vi "DB Select.vi"(6 "Select":enum16{"SelectWithQuery", "SelectWithColumn"}(ring)=enum."SelectWithColumn", 8 "error in (no error)":errorcluster, 9 "SQLTableData":T1, 10 "SQL query":string, 11 "Database in":refnum<class "SQLite Database.lvclass">) -> (0 "error out":errorcluster, 2 "data":string[][](array[string]), 3 "Database out":refnum<class "SQLite Database.lvclass">)   [LabVIEW 2023, in "HardwareAbstractionLayer_LVOOP.lvlib" / "SQLite Database.lvclass"]
uses:
  SQLite Database.lvclass
  SQLite Database.lvclass/SQLite Database.ctl
  <vilib>/addons/database/Connection.llb/Conn Execute.vi
  <vilib>/addons/database/Recordset.llb/Rec Fetch Recordset Data (R).vi
  <vilib>/addons/database/Recordset.llb/Rec Destroy - Connection.vi
  <vilib>/addons/database/NI_Database_API.lvlib
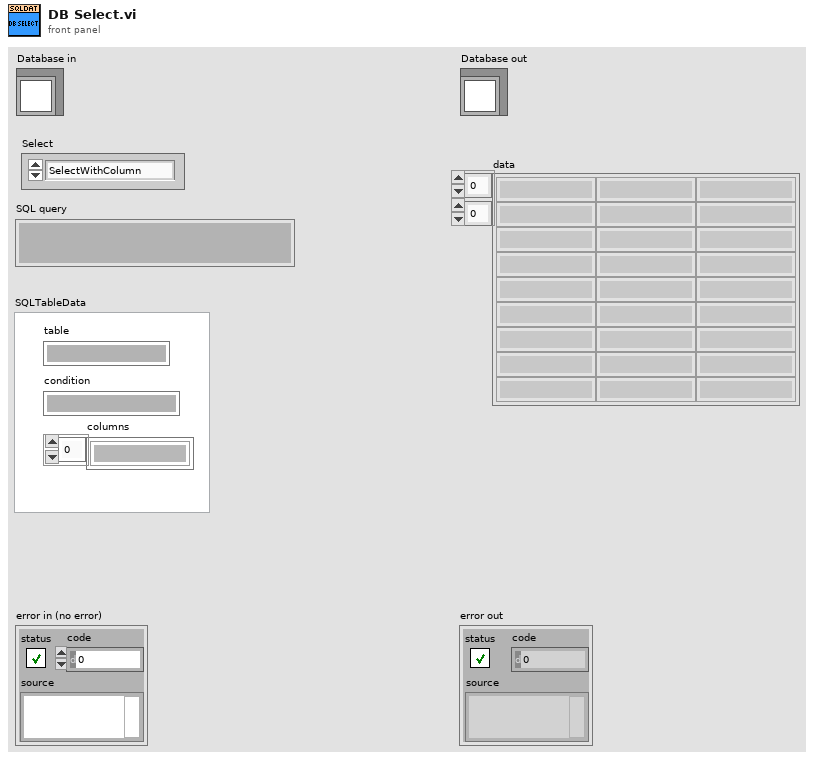
[diagram p1: front panel]
types:
  T1 = cluster{"table":string, "condition":string, "columns":string[]}
  T2 = cluster{"DataSource Name":string, "userID":string, "password":string}
  T3 = typedef "NI_Database_API.lvlib/Conn ObjectReference.ctl" = refnum<k1>
  T4 = typedef "NI_Database_API.lvlib/Rec ObjectReference.ctl" = refnum<k1>
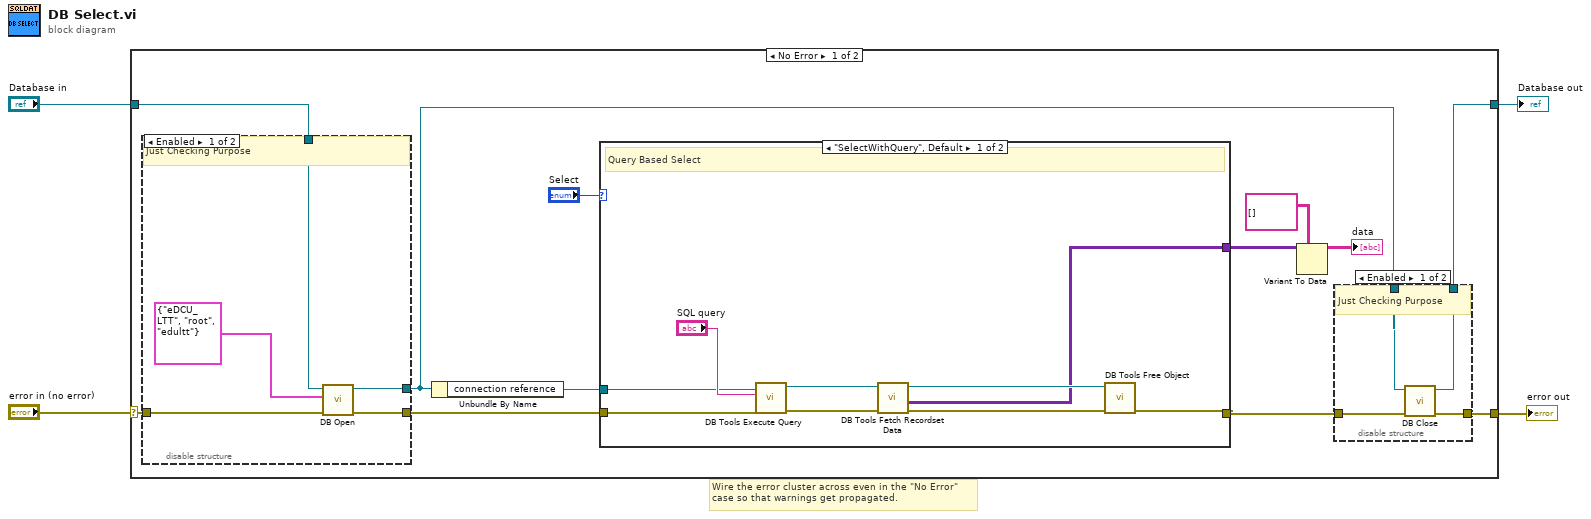
[diagram p0: block diagram]
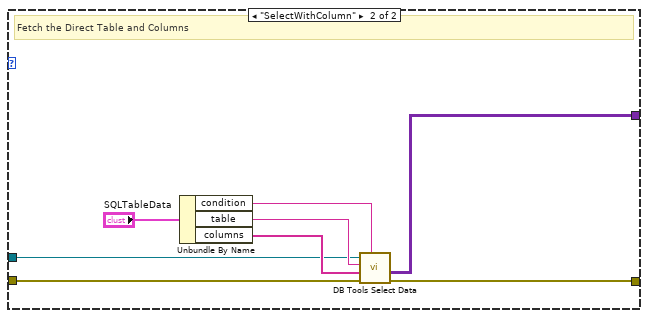
[diagram p4: hidden frame]
diagram:
  # "Wire the error cluster across even in the \"No Error\"\ncase so that warnings get propagated."
  n1 = case shown="No Error" "error in (no error)" {
    selector: "error in (no error)" -> [w11 w47]
    tunnel: [w5 w48] -> w1
    tunnel: "Database in" -> [w12 w48]
    tunnel: [w7 w47] -> w2
    frame No Error {
      n2 = disable-structure shown="Enabled" {
        disable-tunnel: w12 -> [w27 w29]
        disable-tunnel: w11 -> [w25 w28]
        disable-tunnel: [w24 w28] -> w10
        disable-tunnel: [w23 w29] -> w6
        frame Enabled {
          # "Just Checking Purpose"
          n3 = call-dynamic "DB Open.vi"("error in"=w25, "DB"=T2 {"DataSource Name"="eDCU_LTT", "userID"="root", "password"="edultt"}, "Database in"=w27) -> ("error out"=w24:errorcluster, "Database out"=w23:refnum<class "SQLite Database.lvclass">)  [unwired: 7 in]
        }
        frame Disabled {
        }
      }
      n4 = Unbundle By Name(w6) -> ("connection reference"=w9:T3)
      n5 = case shown="\"SelectWithQuery\", Default" "Select" {
        tunnel: w10 -> [w38 w46]
        tunnel: [w35 w45] -> w8
        tunnel: [w32 w44] -> w14
        tunnel: w9 -> [w30 w39]
        frame "SelectWithQuery", Default {
          # "Query Based Select"
          n6 = call-poly <vilib>:"DB Tools Execute Query.vi"("error in (no error)"=w38, "SQL query"="SQL query", "connection reference"=w30) -> ("error out"=w37:errorcluster, "recordset reference"=w33:T4)  [unwired: 5 in]
          n7 = call-poly <vilib>:"DB Tools Fetch Recordset Data.vi"("error in (no error)"=w37, "recordset reference"=w33) -> ("error out"=w36:errorcluster, "recordset data"=w32:variant[][], "recordset reference out"=w34:T4)  [unwired: 3 in]
          n8 = call-poly <vilib>:"DB Tools Free Object.vi"("error in (no error)"=w36, "recordset reference"=w34) -> ("error out"=w35:errorcluster)  [unwired: 8 in, 1 out]
        }
        frame "SelectWithColumn" {
          # "Fetch the Direct Table and Columns"
          n9 = Unbundle By Name("SQLTableData") -> ("condition"=w42:string, "table"=w41:string, "columns"=w40:string[])
          n10 = call <vilib>:"DB Tools Select Data.vi"("condition"=w42, "error in (no error)"=w46, "columns"=w40, "table"=w41, "connection reference"=w39) -> ("error out"=w45:errorcluster, "data"=w44:variant[][])  [unwired: 1 in, 1 out]
        }
      }
      n11 = Variant To Data(type=string[][] [], Variant=w14) -> (data=→"data":string[][])  [unwired: 1 in, 1 out]
      n12 = disable-structure shown="Enabled" {
        disable-tunnel: w8 -> [w20 w22]
        disable-tunnel: [w19 w22] -> w7
        disable-tunnel: w6 -> [w18 w21]
        disable-tunnel: [w17 w21] -> w5
        frame Enabled {
          # "Just Checking Purpose"
          n13 = call-dynamic "DB Close.vi"("error in"=w20, "Database in"=w18) -> ("error out"=w19:errorcluster, "Database out"=w17:refnum<class "SQLite Database.lvclass">)  [unwired: 8 in]
        }
        frame Disabled {
          # "Just Checking Purpose"
        }
      }
    }
    frame Error {
    }
  }
  "error out" <- w2
  "Database out" <- w1
